vi "begin gauss.vi"() -> ()   [LabVIEW 2012, in "LightPipes.lvlib"]
uses:
  LightPipes.lvlib
panel:
  in  "AA":dbl=1.0
  in  "ys":dbl
  in  "xs":dbl
  in  "Path":path=path "C:/Users/Green Beret/Documents/Visual Studio 2012/Projects/LightPipes/LightPipes/lp12src/LabView/images/beam.pgm"
  in  "size_grid":dbl=0.01
  in  "n_grid":i32=256
  in  "R":dbl=0.001
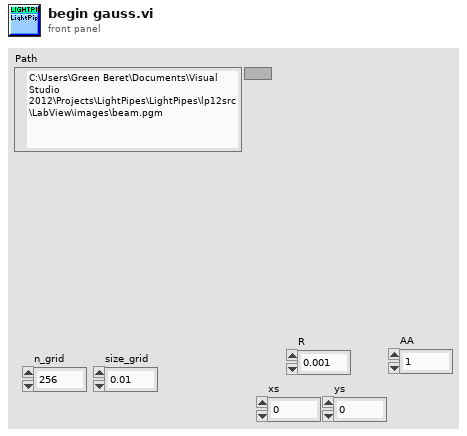
[diagram p1: front panel]
types:
  T1 = cluster{"n_grid":i32, "@dummy control@":i8, "@dummy control@":i8, "@dummy control@":i8, "@dummy control@":i8, "size":dbl, "lambda":dbl, "int1":i32, "int2":i32, "int3":i32, "@dummy control@":i8, "@dummy control@":i8, "@dummy control@":i8, "@dummy control@":i8, "double1":dbl, "double2":dbl, "double3":dbl, "real":u32, "imaginary":u32}
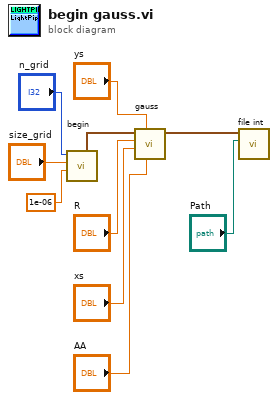
[diagram p0: block diagram]
diagram:
  n1 = call "begin.vi"("lambda"=1e-06, "size_grid"="size_grid", "n_grid"="n_grid") -> ("field out"=w10:T1)  [unwired: 8 in]
  n2 = call "gauss.vi"("AA"="AA", "ys"="ys", "xs"="xs", "R"="R", "field"=w10) -> ("field out"=w1:T1)  [unwired: 6 in]
  n3 = call "file int.vi"("Path in"="Path", "field"=w1) -> ()  [unwired: 9 in, 1 out]
